vi "VI Tree.vi"   [LabVIEW 2012, in "Agilent PSG MXG Series.lvlib"]
doc: "This is the instrument driver for the Agilent PSG MXG Series. The VI Tree displays all the user-callable VIs of the instrument driver in an organized table."
uses:
  <instrlib>/Agilent PSG MXG Series/Agilent PSG MXG Series.lvlib
  <instrlib>/Agilent PSG MXG Series/Public/Configure/Configure Sweep (List).vi
  <instrlib>/Agilent PSG MXG Series/Public/Configure/Modulation/Configure Modulation (Amplitude).vi
  <instrlib>/Agilent PSG MXG Series/Public/Configure/Modulation/Configure Modulation Waveform Advanced (Swept-Sine).vi
  <instrlib>/Agilent PSG MXG Series/Public/Configure/Modulation/Configure Modulation Waveform (Noise).vi
panel:
  # "(c) 2012 National Instruments.  ALL RIGHTS RESERVED."
  # "SEE DIAGRAM\nFOR VI TREE."
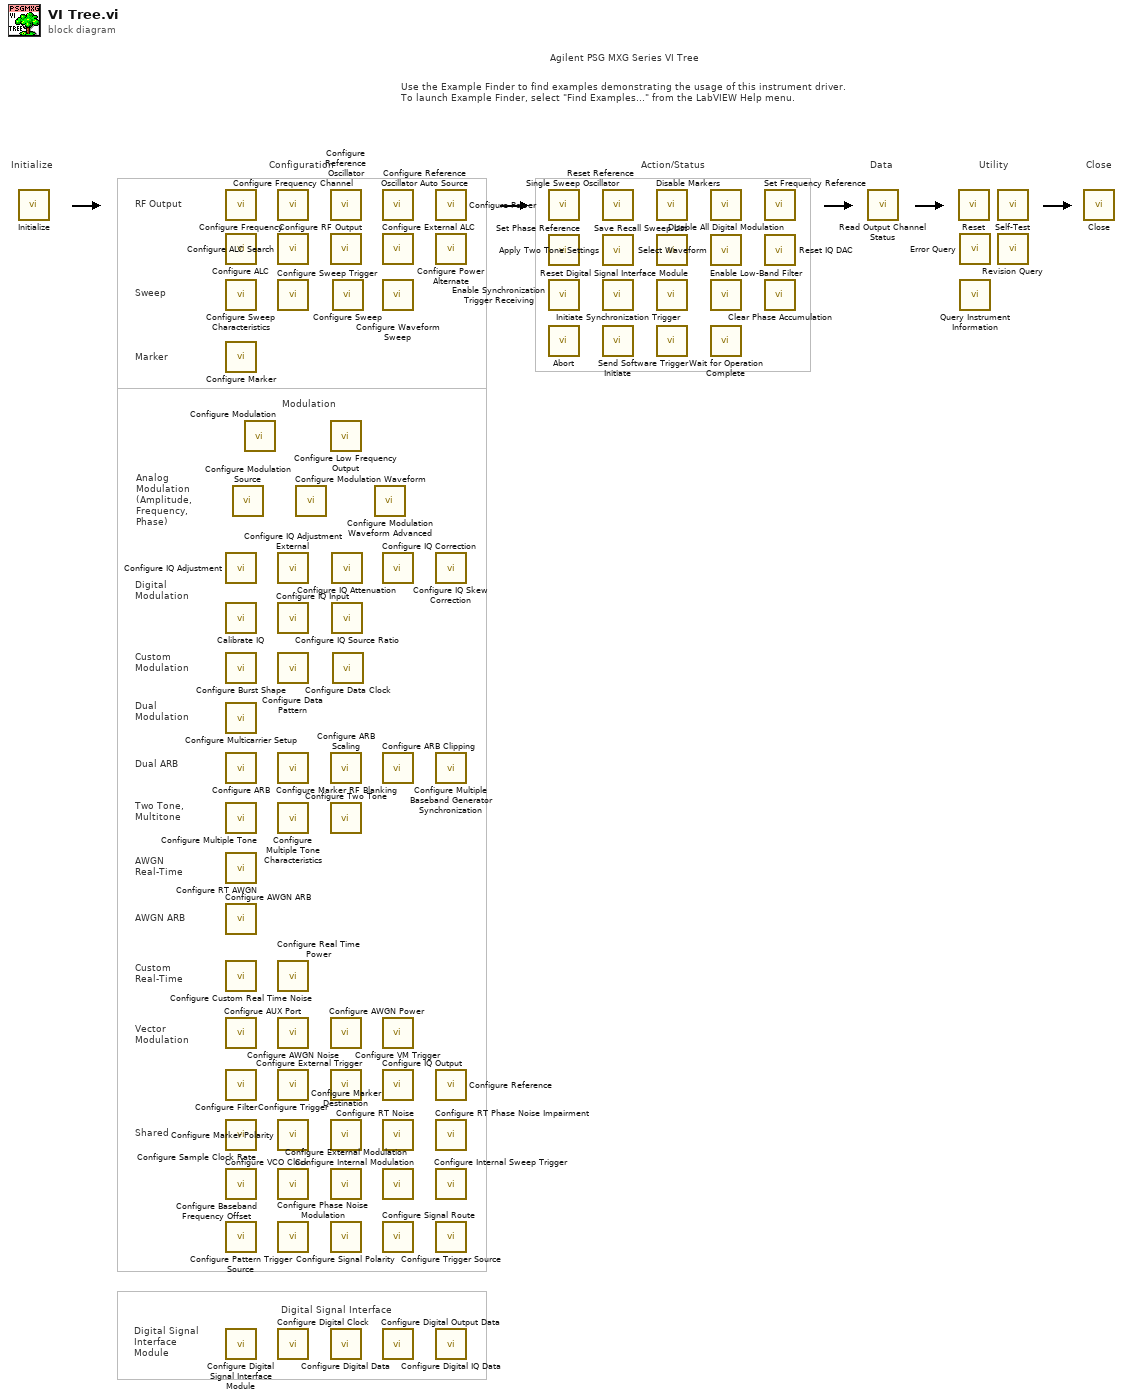
[diagram p0: block diagram]
diagram:
  # "Data"
  # "Vector\nModulation"
  # "Custom\nReal-Time"
  # "AWGN ARB"
  # "Digital Signal Interface"
  # "Marker"
  # "Digital Signal\nInterface\nModule"
  # "AWGN\nReal-Time"
  # "Shared"
  # "Two Tone,\nMultitone"
  # "Dual ARB"
  # "Dual\nModulation"
  # "Custom\nModulation"
  # "Digital\nModulation"
  # "Analog\nModulation\n(Amplitude,\nFrequency,\nPhase)"
  # "Sweep"
  # "RF Output"
  # "Modulation"
  # "Agilent PSG MXG Series VI Tree"
  # "Use the Example Finder to find examples demonstrating the usage of this instrument driver.\nTo launch Example Finder, select \"Find Examples...\" from the LabVIEW Help menu."
  # "Configuration"
  # "Utility"
  # "Action/Status"
  # "Close"
  # "Initialize"
  n1 = call <instrlib>:"Initialize.vi"() -> ()  [unwired: 10 in, 2 out]
  n2 = call <instrlib>:"Configure Frequency.vi"() -> ()  [unwired: 14 in, 2 out]
  n3 = call <instrlib>:"Configure ALC.vi"() -> ()  [unwired: 14 in, 2 out]
  n4 = call <instrlib>:"Configure Sweep Characteristics.vi"() -> ()  [unwired: 14 in, 2 out]
  n5 = call <instrlib>:"Configure Marker.vi"() -> ()  [unwired: 14 in, 2 out]
  n6 = call <instrlib>:"Configure IQ Adjustment.vi"() -> ()  [unwired: 14 in, 2 out]
  n7 = call <instrlib>:"Calibrate IQ.vi"() -> ()  [unwired: 10 in, 2 out]
  n8 = call <instrlib>:"Configure Burst Shape.vi"() -> ()  [unwired: 14 in, 2 out]
  n9 = call <instrlib>:"Configure Multicarrier Setup.vi"() -> ()  [unwired: 14 in, 2 out]
  n10 = call <instrlib>:"Configure ARB.vi"() -> ()  [unwired: 10 in, 2 out]
  n11 = call <instrlib>:"Configure Multiple Tone.vi"() -> ()  [unwired: 14 in, 2 out]
  n12 = call <instrlib>:"Configure RT AWGN.vi"() -> ()  [unwired: 10 in, 2 out]
  n13 = call <instrlib>:"Configure AWGN ARB.vi"() -> ()  [unwired: 10 in, 2 out]
  n14 = call <instrlib>:"Configure Custom Real Time Noise.vi"() -> ()  [unwired: 10 in, 2 out]
  n15 = call <instrlib>:"Configrue AUX Port.vi"() -> ()  [unwired: 10 in, 2 out]
  n16 = call <instrlib>:"Configure Filter.vi"() -> ()  [unwired: 14 in, 2 out]
  n17 = call <instrlib>:"Configure Sample Clock Rate.vi"() -> ()  [unwired: 10 in, 2 out]
  n18 = call <instrlib>:"Configure Baseband Frequency Offset.vi"() -> ()  [unwired: 10 in, 2 out]
  n19 = call <instrlib>:"Configure Pattern Trigger Source.vi"() -> ()  [unwired: 10 in, 2 out]
  n20 = call <instrlib>:"Configure Digital Signal Interface Module.vi"() -> ()  [unwired: 10 in, 2 out]
  n21 = call <instrlib>:"Configure Modulation Source.vi"() -> ()  [unwired: 14 in, 2 out]
  n22 = call-poly <instrlib>:"Configure Modulation.vi"() -> ()  [unwired: 14 in, 2 out]
  n23 = call <instrlib>:"Configure Frequency Channel.vi"() -> ()  [unwired: 10 in, 2 out]
  n24 = call <instrlib>:"Configure ALC Search.vi"() -> ()  [unwired: 14 in, 2 out]
  n25 = call <instrlib>:"Configure Sweep Trigger.vi"() -> ()  [unwired: 14 in, 2 out]
  n26 = call <instrlib>:"Configure IQ Adjustment External.vi"() -> ()  [unwired: 14 in, 2 out]
  n27 = call <instrlib>:"Configure IQ Input.vi"() -> ()  [unwired: 10 in, 2 out]
  n28 = call <instrlib>:"Configure Data Pattern.vi"() -> ()  [unwired: 10 in, 2 out]
  n29 = call <instrlib>:"Configure Marker RF Blanking.vi"() -> ()  [unwired: 10 in, 2 out]
  n30 = call <instrlib>:"Configure Multiple Tone Characteristics.vi"() -> ()  [unwired: 10 in, 2 out]
  n31 = call <instrlib>:"Configure Real Time Power.vi"() -> ()  [unwired: 10 in, 2 out]
  n32 = call <instrlib>:"Configure AWGN Noise.vi"() -> ()  [unwired: 14 in, 2 out]
  n33 = call <instrlib>:"Configure Trigger.vi"() -> ()  [unwired: 14 in, 2 out]
  n34 = call <instrlib>:"Configure Marker Polarity.vi"() -> ()  [unwired: 10 in, 2 out]
  n35 = call <instrlib>:"Configure VCO Clock.vi"() -> ()  [unwired: 10 in, 2 out]
  n36 = call <instrlib>:"Configure Phase Noise Modulation.vi"() -> ()  [unwired: 10 in, 2 out]
  n37 = call <instrlib>:"Configure Digital Clock.vi"() -> ()  [unwired: 14 in, 2 out]
  n38 = call-poly <instrlib>:"Configure Modulation Waveform.vi"() -> ()  [unwired: 10 in, 2 out]
  n39 = call <instrlib>:"Configure Reference Oscillator.vi"() -> ()  [unwired: 10 in, 2 out]
  n40 = call <instrlib>:"Configure RF Output.vi"() -> ()  [unwired: 10 in, 2 out]
  n41 = call <instrlib>:"Configure Low Frequency Output.vi"() -> ()  [unwired: 14 in, 2 out]
  n42 = call <instrlib>:"Configure ARB Scaling.vi"() -> ()  [unwired: 10 in, 2 out]
  n43 = call <instrlib>:"Configure Two Tone.vi"() -> ()  [unwired: 10 in, 2 out]
  n44 = call <instrlib>:"Configure AWGN Power.vi"() -> ()  [unwired: 10 in, 2 out]
  n45 = call <instrlib>:"Configure External Trigger.vi"() -> ()  [unwired: 10 in, 2 out]
  n46 = call <instrlib>:"Configure Marker Destination.vi"() -> ()  [unwired: 10 in, 2 out]
  n47 = call <instrlib>:"Configure External Modulation.vi"() -> ()  [unwired: 10 in, 2 out]
  n48 = call <instrlib>:"Configure Signal Polarity.vi"() -> ()  [unwired: 10 in, 2 out]
  n49 = call <instrlib>:"Configure Digital Data.vi"() -> ()  [unwired: 14 in, 2 out]
  n50 = call <instrlib>:"Configure IQ Attenuation.vi"() -> ()  [unwired: 10 in, 2 out]
  n51 = call <instrlib>:"Configure IQ Source Ratio.vi"() -> ()  [unwired: 10 in, 2 out]
  n52 = call-poly <instrlib>:"Configure Sweep.vi"() -> ()  [unwired: 14 in, 2 out]
  n53 = call <instrlib>:"Configure Data Clock.vi"() -> ()  [unwired: 10 in, 2 out]
  n54 = call-poly <instrlib>:"Configure Modulation Waveform Advanced.vi"() -> ()  [unwired: 14 in, 2 out]
  n55 = call <instrlib>:"Configure Reference Oscillator Auto Source.vi"() -> ()  [unwired: 10 in, 2 out]
  n56 = call <instrlib>:"Configure External ALC.vi"() -> ()  [unwired: 10 in, 2 out]
  n57 = call <instrlib>:"Configure Waveform Sweep.vi"() -> ()  [unwired: 10 in, 2 out]
  n58 = call <instrlib>:"Configure IQ Correction.vi"() -> ()  [unwired: 10 in, 2 out]
  n59 = call <instrlib>:"Configure ARB Clipping.vi"() -> ()  [unwired: 10 in, 2 out]
  n60 = call <instrlib>:"Configure VM Trigger.vi"() -> ()  [unwired: 10 in, 2 out]
  n61 = call <instrlib>:"Configure IQ Output.vi"() -> ()  [unwired: 14 in, 2 out]
  n62 = call <instrlib>:"Configure RT Noise.vi"() -> ()  [unwired: 14 in, 2 out]
  n63 = call <instrlib>:"Configure Internal Modulation.vi"() -> ()  [unwired: 14 in, 2 out]
  n64 = call <instrlib>:"Configure Signal Route.vi"() -> ()  [unwired: 10 in, 2 out]
  n65 = call <instrlib>:"Configure Digital Output Data.vi"() -> ()  [unwired: 10 in, 2 out]
  n66 = call <instrlib>:"Configure Power.vi"() -> ()  [unwired: 14 in, 2 out]
  n67 = call <instrlib>:"Configure Power Alternate.vi"() -> ()  [unwired: 10 in, 2 out]
  n68 = call <instrlib>:"Configure IQ Skew Correction.vi"() -> ()  [unwired: 10 in, 2 out]
  n69 = call <instrlib>:"Configure Multiple Baseband Generator Synchronization.vi"() -> ()  [unwired: 10 in, 2 out]
  n70 = call <instrlib>:"Configure Reference.vi"() -> ()  [unwired: 10 in, 2 out]
  n71 = call <instrlib>:"Configure RT Phase Noise Impairment.vi"() -> ()  [unwired: 10 in, 2 out]
  n72 = call <instrlib>:"Configure Internal Sweep Trigger.vi"() -> ()  [unwired: 14 in, 2 out]
  n73 = call <instrlib>:"Configure Trigger Source.vi"() -> ()  [unwired: 10 in, 2 out]
  n74 = call <instrlib>:"Configure Digital IQ Data.vi"() -> ()  [unwired: 14 in, 2 out]
  n75 = call <instrlib>:"Single Sweep.vi"() -> ()  [unwired: 10 in, 2 out]
  n76 = call <instrlib>:"Set Phase Reference.vi"() -> ()  [unwired: 10 in, 2 out]
  n77 = call <instrlib>:"Enable Synchronization Trigger Receiving.vi"() -> ()  [unwired: 10 in, 2 out]
  n78 = call <instrlib>:"Abort.vi"() -> ()  [unwired: 10 in, 2 out]
  n79 = call <instrlib>:"Reset Reference Oscillator.vi"() -> ()  [unwired: 10 in, 2 out]
  n80 = call <instrlib>:"Apply Two Tone Settings.vi"() -> ()  [unwired: 10 in, 2 out]
  n81 = call <instrlib>:"Initiate Synchronization Trigger.vi"() -> ()  [unwired: 10 in, 2 out]
  n82 = call <instrlib>:"Initiate.vi"() -> ()  [unwired: 10 in, 2 out]
  n83 = call <instrlib>:"Disable Markers.vi"() -> ()  [unwired: 10 in, 2 out]
  n84 = call <instrlib>:"Save Recall Sweep List.vi"() -> ()  [unwired: 10 in, 2 out]
  n85 = call <instrlib>:"Reset Digital Signal Interface Module.vi"() -> ()  [unwired: 10 in, 2 out]
  n86 = call <instrlib>:"Send Software Trigger.vi"() -> ()  [unwired: 10 in, 2 out]
  n87 = call <instrlib>:"Disable All Digital Modulation.vi"() -> ()  [unwired: 10 in, 2 out]
  n88 = call <instrlib>:"Select Waveform.vi"() -> ()  [unwired: 10 in, 2 out]
  n89 = call <instrlib>:"Enable Low-Band Filter.vi"() -> ()  [unwired: 10 in, 2 out]
  n90 = call <instrlib>:"Wait for Operation Complete.vi"() -> ()  [unwired: 10 in, 2 out]
  n91 = call <instrlib>:"Set Frequency Reference.vi"() -> ()  [unwired: 10 in, 2 out]
  n92 = call <instrlib>:"Reset IQ DAC.vi"() -> ()  [unwired: 10 in, 2 out]
  n93 = call <instrlib>:"Clear Phase Accumulation.vi"() -> ()  [unwired: 10 in, 2 out]
  n94 = call <instrlib>:"Read Output Channel Status.vi"() -> ()  [unwired: 9 in, 3 out]
  n95 = call <instrlib>:"Reset.vi"() -> ()  [unwired: 10 in, 2 out]
  n96 = call <instrlib>:"Error Query.vi"() -> ()  [unwired: 8 in, 4 out]
  n97 = call <instrlib>:"Query Instrument Information.vi"() -> ()  [unwired: 8 in, 8 out]
  n98 = call <instrlib>:"Self-Test.vi"() -> ()  [unwired: 8 in, 4 out]
  n99 = call <instrlib>:"Revision Query.vi"() -> ()  [unwired: 8 in, 4 out]
  n100 = call <instrlib>:"Close.vi"() -> ()  [unwired: 11 in, 1 out]
